vi "ADO Connection Drop Table.vi"(8 "error in (no error)":errorcluster caption="错误输入（无错误）", 9 "Table":string, 11 "Database Connection 输入":refnum<class "Database Connection.lvclass"> caption="DNL_LabVIEW Object in") -> (0 "error out":errorcluster caption="错误输出", 3 "Database Connection 输出":refnum<class "Database Connection.lvclass"> caption="DNL_LabVIEW Object out")   [LabVIEW 2011, in "Database Connection.lvclass"]
uses:
  Database Connection.lvclass
  Recordset/Database Recordset.lvclass
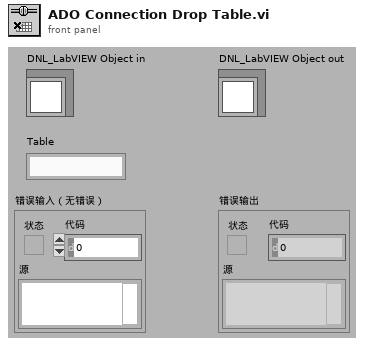
[diagram p1: front panel]
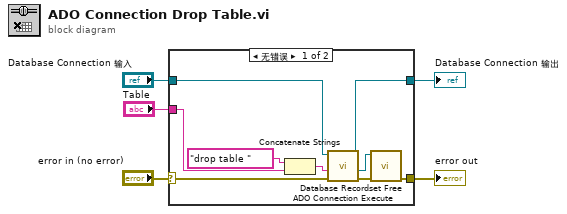
[diagram p0: block diagram]
diagram:
  n1 = case shown="无错误" "error in (no error)" {
    selector: "error in (no error)" -> [w9 w16]
    tunnel: [w8 w16] -> w4
    tunnel: [w6 w15] -> w2
    tunnel: "Database Connection 输入" -> [w11 w15]
    tunnel: "Table" -> [w13 _]
    frame No Error {
      n2 = Concatenate Strings("drop table ", w13) -> (w12:string)
      n3 = call "ADO Connection Execute.vi"("error in (no error)"=w9, "CommandText"=w12, "Database Connection 输入"=w11) -> ("error out"=w10:errorcluster, "Database Recordset输出"=w7:refnum<class "Database Recordset.lvclass">, "Database Connection 输出"=w6:refnum<class "Database Connection.lvclass">)  [unwired: 6 in]
      n4 = call "Database Recordset Free.vi"("error in (no error)"=w10, "Database Recordset 输入"=w7) -> ("error out"=w8:errorcluster)  [unwired: 9 in]
    }
    frame Error {
    }
  }
  "error out" <- w4
  "Database Connection 输出" <- w2
